vi "Get Data Type Object by Index.vi"(8 "error in (no error)":errorcluster, 10 "Index":i32, 11 "DataGrid Config in":refnum<class "DataGrid Config.lvclass">) -> (0 "error out":errorcluster, 2 "Data Type Object":refnum<class "Generic Data Type.lvclass">, 3 "DataGrid Config (dup)":refnum<class "DataGrid Config.lvclass">)   [LabVIEW 2018, in "DataGrid Config.lvclass"]
uses:
  DataGrid Config.lvclass
  Data Type Classes/Generic/Generic Data Type.lvclass
  DataGrid Config.lvclass/DataGrid Config.ctl
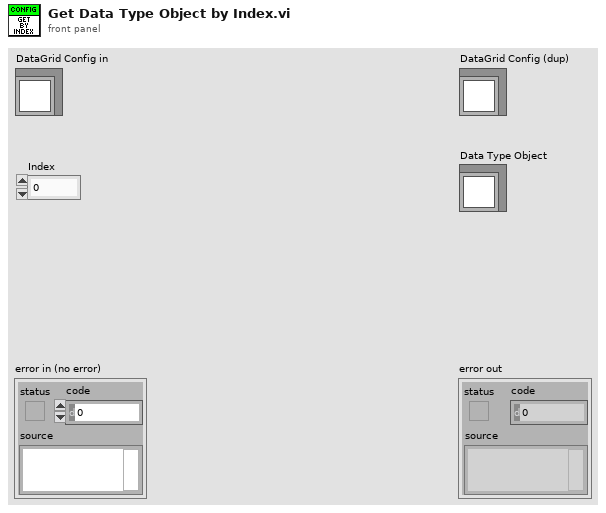
[diagram p1: front panel]
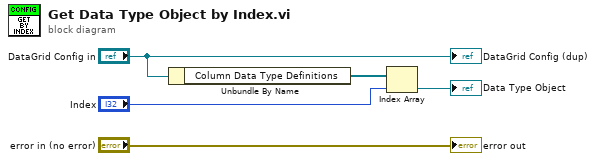
[diagram p0: block diagram]
diagram:
  n1 = Unbundle By Name("DataGrid Config in") -> ("Column Data Type Definitions"=w4:refnum<class "Generic Data Type.lvclass">[])
  n2 = Index Array(array=w4, index="Index") -> (element=→"Data Type Object":refnum<class "Generic Data Type.lvclass">)
  "error out" <- "error in (no error)"
  "DataGrid Config (dup)" <- "DataGrid Config in"
